vi "Test Time Measurement Runner.vi"() -> ()   [LabVIEW 2018]
panel:
  out "VI Tester Testing time (seconds)":dbl
  out "ICov Testing time (seconds)":dbl
  out "Caraya Testing time (seconds)":dbl
  out "UTF Testing time (seconds)":dbl
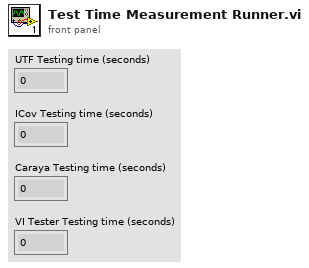
[diagram p1: front panel]
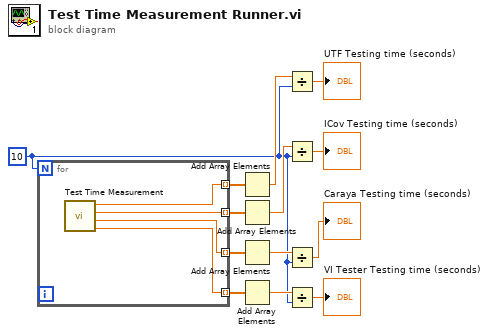
[diagram p0: block diagram]
diagram:
  w5 = 10
  n1 = for {
    N: w5 -> [_]
    tunnel: [w17] -> w13 mode=indexing
    tunnel: [w16] -> w12 mode=indexing
    tunnel: [w15] -> w11 mode=indexing
    tunnel: [w14] -> w10 mode=indexing
    n2 = call "Test Time Measurement.vi"() -> ("VI Tester Testing time (seconds)"=w14:dbl, "Caraya Testing time (seconds)"=w16:dbl, "ICov Testing time (seconds)"=w15:dbl, "UTF Testing time (seconds)"=w17:dbl)  [unwired: 8 in]
  }
  n3 = Add Array Elements(numeric array=w13) -> (sum=w9:dbl)
  n4 = Add Array Elements(numeric array=w11) -> (sum=w7:dbl)
  n5 = Add Array Elements(numeric array=w12) -> (sum=w8:dbl)
  n6 = Add Array Elements(numeric array=w10) -> (sum=w6:dbl)
  n7 = Divide(x=w9, y=w5) -> (x/y=→"UTF Testing time (seconds)":dbl)
  n8 = Divide(x=w7, y=w5) -> (x/y=→"ICov Testing time (seconds)":dbl)
  n9 = Divide(x=w8, y=w5) -> (x/y=→"Caraya Testing time (seconds)":dbl)
  n10 = Divide(x=w6, y=w5) -> (x/y=→"VI Tester Testing time (seconds)":dbl)
